vi "CM-Channel Names to Indices.vi"(0 "IO Channels":string[](array[string]), 2 "IO Type":T1=enum."Digital Outputs", 11 "error in (no error)":errorcluster) -> (4 "Indices":i32[](array[numeric]), 15 "error out":errorcluster)   [LabVIEW 2020]
uses:
  Type Defs/CM-IO Type.ctl
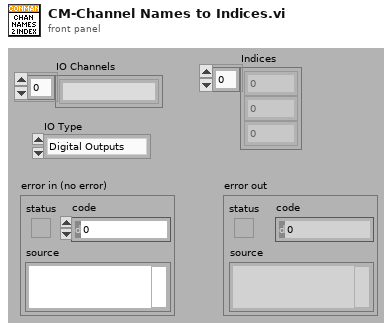
[diagram p1: front panel]
types:
  T1 = typedef "CM-IO Type.ctl" = enum16{"Analog Outputs", "Analog Inputs", "Digital Outputs", "Digital Inputs"}
  T2 = typedef "PXI-Device Spec.ctl" = cluster{"Slot":i32, "ProductType":string, "NumAO":i32, "NumAI":i32, "Device Name":string}
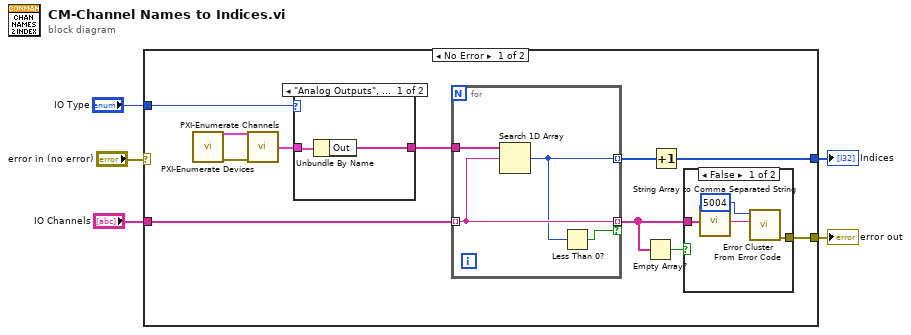
[diagram p0: block diagram]
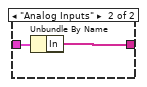
[diagram p3: hidden frame]
diagram:
  n1 = case shown="No Error" "error in (no error)" {
    selector: "error in (no error)" -> [_ w29]
    tunnel: [w7 w29] -> w4
    tunnel: "IO Type" -> [w13 _]
    tunnel: "IO Channels" -> [w11 _]
    tunnel: [w6 _] -> w1
    frame No Error {
      n2 = call "PXI-Enumerate Devices.vi"() -> ("Devices"=w16:T2[], "error out"=w15:errorcluster)  [unwired: 14 in]
      n3 = call "PXI-Enumerate Channels.vi"("Devices"=w16, "error in (no error)"=w15) -> ("Channels (1D)"=w14:cluster{"Out":string[], "In":string[]})  [unwired: 11 in, 2 out]
      n4 = case shown="\"Analog Outputs\", Default" w13 {
        tunnel: w14 -> [w26 w28]
        tunnel: [w25 w27] -> w12
        frame "Analog Outputs", Default {
          n5 = Unbundle By Name(w26) -> ("Out"=w25:string[])
        }
        frame "Analog Inputs" {
          n6 = Unbundle By Name(w28) -> ("In"=w27:string[])
        }
      }
      n7 = for {
        tunnel: w12 -> [w24]
        tunnel: w11 -> [w23] mode=indexing
        tunnel: [w22] -> w10 mode=indexing
        tunnel: [w23] -> w8 mode=indexing if=w21
        n8 = Search 1D Array(1D array=w24, element=w23) -> (index of element=w22:i32)  [unwired: 1 in]
        n9 = Less Than 0?(x=w22) -> (x < 0?=w21:bool)
      }
      n10 = Empty Array?(array=w8) -> (empty?=w9:bool)
      n11 = Increment(x=w10) -> (x+1=w6:i32[])
      n12 = case shown="False" w9 {
        tunnel: w8 -> [w18 _]
        tunnel: [w17 _] -> w7
        frame False {
          n13 = call "String Array to Comma Separated String.vi"("String Array"=w18) -> ("comma separated string"=w19:string)
          n14 = call <vilib>:"Error Cluster From Error Code.vi"("error message (\"\")"=w19, "error code (0)"=5004) -> ("error out"=w17:errorcluster)  [unwired: 7 in]
        }
        frame True {
        }
      }
    }
    frame Error {
    }
  }
  "error out" <- w4
  "Indices" <- w1
